vi "ManipActuateGripper.vi"(3 "Parameter String":string) -> (0 "error out":errorcluster, 1 "Advance Trigger":bool)   [LabVIEW 2020]
doc: "This VI commands the gripper to open or close during a systems check\n\nParameters:\nDecides open or closed state of the gripper (\"open\" or \"close\")"
uses:
  SafeParser_String.vi
  GlobalAutonomous.vi
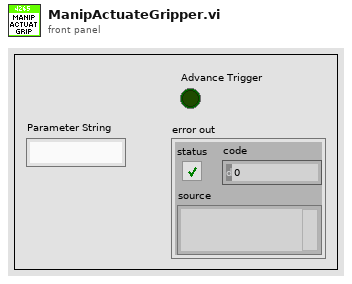
[diagram p1: front panel]
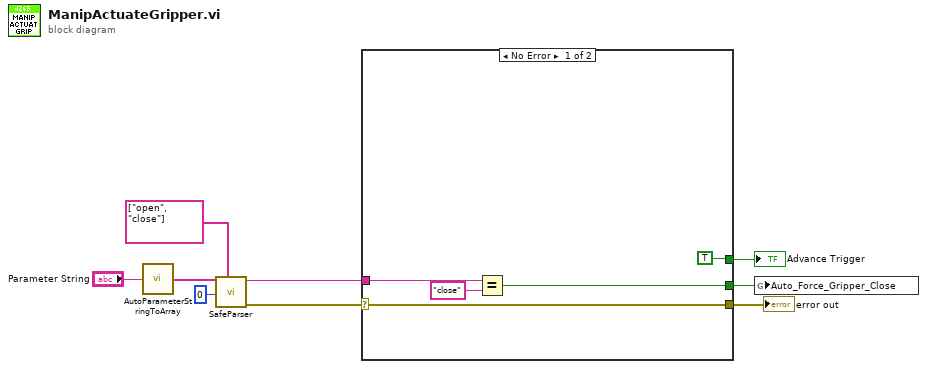
[diagram p0: block diagram]
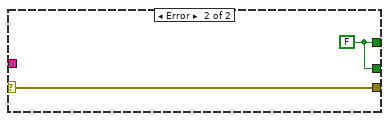
[diagram p2: hidden frame]
diagram:
  n1 = call "AutoParameterStringToArray.vi"("Parameter String"="Parameter String") -> ("Parsed Parameters"=w7:string[])
  n2 = call-poly "SafeParser.vi"("Allowed Values"=string[] ["open", "close"], "Array Index"=0 ("Parameter Index"), "String Array"=w7) -> ("Error Out"=w5:errorcluster, "Typecast Value"=w3:string)  [unwired: 7 in]
  n3 = case shown="No Error" w5 {
    selector: w5 -> [w14 w16]
    tunnel: [w12 w15] -> w2
    tunnel: [w14 w16] -> w4
    tunnel: w3 -> [w13 _]
    tunnel: [TRUE w15] -> w1
    frame No Error {
      n4 = Equal?(x=w13, y="close") -> (x = y?=w12:bool)
    }
    frame Error {
      w15 = FALSE
    }
  }
  "Advance Trigger" <- w1
  "error out" <- w4
  n5 = global write "GlobalAutonomous.vi" "Auto_Force_Gripper_Close"(w2) -> ()
